vi "Uniform PDF.vi"(9 "xmax":dbl=1.0, 10 "xmin":dbl, 11 "x":dbl) -> (0 "error":i32, 3 "pdf(x)":dbl=1.0)   [LabVIEW 2020, in "NI_Gmath.lvlib"]
doc: "Computes the continuous probability density function (PDF) of various distributions. You must manually select the polymorphic instance to use."
uses:
  NI_Gmath.lvlib
  st_error_code.ctl
panel:
  # "Uniform PDF"
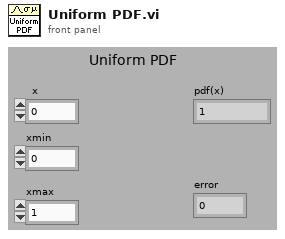
[diagram p1: front panel]
types:
  T1 = typedef "NI_Gmath.lvlib/st_error_code.ctl" = i32
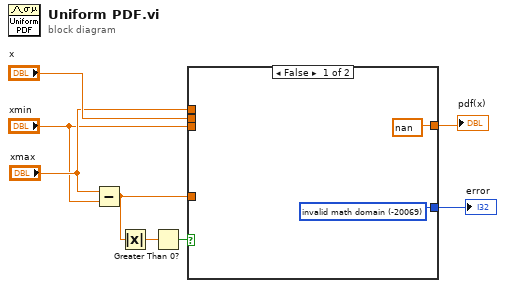
[diagram p0: block diagram]
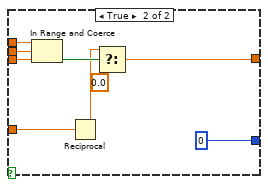
[diagram p2: hidden frame]
diagram:
  n1 = Subtract(x="xmax", y="xmin") -> (x-y=w4:dbl)
  n2 = Absolute Value(x=w4) -> (abs(x)=w5:dbl)
  n3 = Greater Than 0?(x=w5) -> (x > 0?=w3:bool)
  n4 = case shown="False" w3 {
    tunnel: "x" -> [_ w19]
    tunnel: "xmax" -> [_ w17]
    tunnel: "xmin" -> [_ w16]
    tunnel: w4 -> [_ w13]
    tunnel: [nan w12] -> w2
    tunnel: [w9 0] -> w1
    frame False {
      w9 = T1 -20069 items=["invalid math domain"=-20069, "Fourier interpolation size m >= n"=-20070, "empty array"=-20003] ("stat interp error code")
    }
    frame True {
      n5 = In Range and Coerce(upper limit=w17, x=w19, lower limit=w16) -> (In Range?=w18:bool)  [unwired: 1 out]
      n6 = Reciprocal(x=w13) -> (1/x=w15:dbl)
      n7 = Select(t=w15, s=w18, f=0.0) -> (s? t:f=w12:dbl)
    }
  }
  "pdf(x)" <- w2
  "error" <- w1
